vi "Column Averager.vi"(1 "Depth Values":dbl[][](array[numeric])) -> (0 "Column Averages":dbl[](array[numeric]))   [LabVIEW 2018]
uses:
  <vilib>/Analysis/baseanly.llb/Mean (DBL).vi
  f516c154-24af-460a-a059-2a37528503fd.vi
  f516c154-24af-460a-a059-2a37528503fd.vi/a82c35f6-fe05-456a-9ce9-2255a9b63c38.vi
  <vilib>/Analysis/NI_AALBase.lvlib
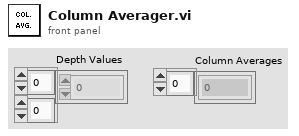
[diagram p1: front panel]
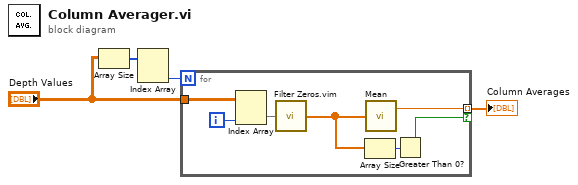
[diagram p0: block diagram]
diagram:
  n1 = Array Size(array="Depth Values") -> (size(s)=w2:i32[])
  n2 = Index Array(array=w2) -> (element #2=w1:i32)  [unwired: 2 in, 1 out]
  n3 = for {
    N: w1 -> [_]
    tunnel: "Depth Values" -> [w11]
    tunnel: [w9] -> w4 mode=indexing if=w5
    i -> [w10]
    n4 = Index Array(array=w11, index (col)=w10) -> (element=w8:dbl[])  [unwired: 1 in]
    n5 = call "Filter Zeros.vim"("Array"=w8) -> ("Array Out"=w7:dbl[])  [unwired: 14 in]
    n6 = Array Size(array=w7) -> (size(s)=w6:i32)
    n7 = call-poly <vilib>:"Mean.vi"("X"=w7) -> ("mean"=w9:dbl)  [unwired: 1 out]
    n8 = Greater Than 0?(x=w6) -> (x > 0?=w5:bool)
  }
  "Column Averages" <- w4
